vi "set Keyword.vi"(8 "error in (no error)":errorcluster, 9 "keyword":string[](array[string]), 10 "keyword index":i32, 11 "ScintillaNET in":refnum<class "ScintillaNET.lvclass">) -> (0 "error out":errorcluster, 3 "ScintillaNET out":refnum<class "ScintillaNET.lvclass">)   [LabVIEW 2018, in "ScintillaNET.lvclass"]
uses:
  ScintillaNET.lvclass
  ScintillaNET.lvclass/ScintillaNET.ctl
  D:/project/hobby/LF2R/LabVIEW/source/ScintillaNET/dll/ScintillaNET.dll
  dll/ScintillaNET.dll
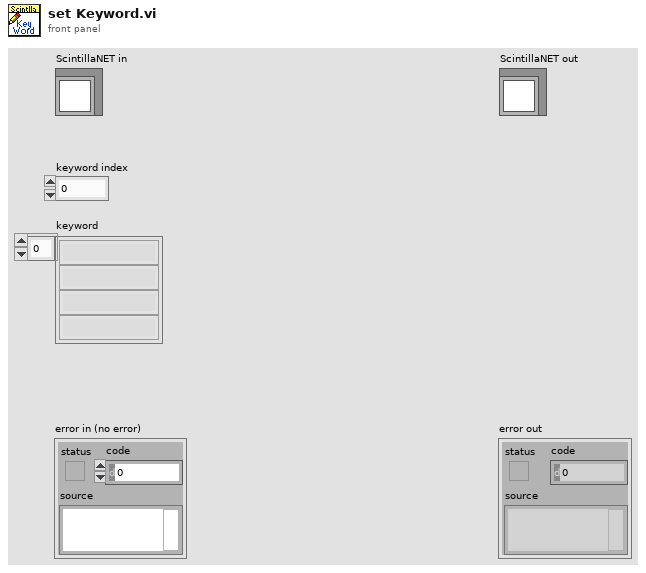
[diagram p1: front panel]
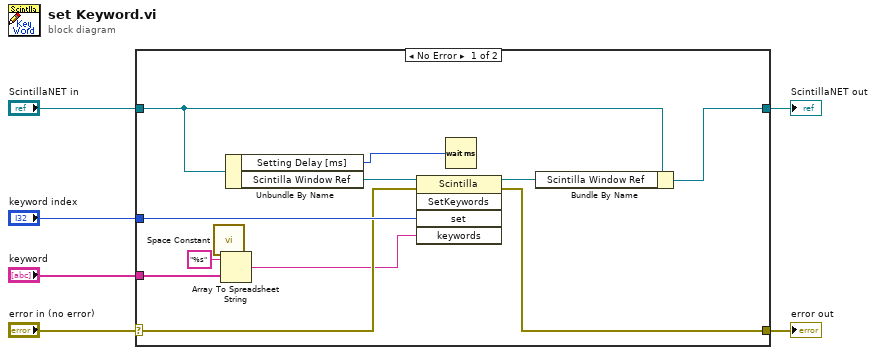
[diagram p0: block diagram]
diagram:
  n1 = case shown="No Error" "error in (no error)" {
    selector: "error in (no error)" -> [w13 w20]
    tunnel: [w12 w20] -> w5
    tunnel: [w17 w19] -> w3
    tunnel: "ScintillaNET in" -> [w18 w19]
    tunnel: "keyword index" -> [w14 _]
    tunnel: "keyword" -> [w11 _]
    frame No Error {
      n2 = call <vilib>:"Space Constant.vi"() -> ("String"=w10:string)
      n3 = Array To Spreadsheet String(delimiter (Tab)=w10, array=w11, 3:"%s" ("format string")) -> (spreadsheet string=w8:string)
      n4 = Unbundle By Name(w18) -> ("Setting Delay [ms]"=w7:u32, "Scintilla Window Ref"=w16:refnum<k24>)
      n5 = invoke class="Scintilla" method="SetKeywords"(reference=w16, error in=w13, "set"=w14, "keywords"=w8) -> (reference out=w15:refnum<k24>, error out=w12:errorcluster)  [unwired: 1 in, 3 out]
      n6 = Wait (ms)(milliseconds to wait=w7) -> ()  [unwired: 1 out]
      n7 = Bundle By Name(cluster=w18, "Scintilla Window Ref"=w15) -> (w17:refnum<class "ScintillaNET.lvclass">)
    }
    frame Error {
    }
  }
  "error out" <- w5
  "ScintillaNET out" <- w3
